vi "one plot adjustable to another.vi"(6 "country index":u16, 7 "SA data":T1, 8 "Countries (in)":string[](array[string]), 9 "US data":T1, 10 "deaths CSV":string[][](array[string]), 11 "cases CSV":string[][](array[string])) -> ()   [LabVIEW 2019]
panel:
  out "XY Graph":T2(graph)
  in  "Country 2":u16(ring) items=["Afghanistan", "Albania", "Algeria", "Andorra", "Angola", "Antigua and Barbuda", "Argentina", "Armenia", "Australia, Australian Capital Territory", "Australia, New South Wales", "Australia, Northern Territory", "Australia, Queensland", "Australia, South Australia", "Australia, Tasmania", "Australia, Victoria", "Australia, Western Australia", "Austria", "Azerbaijan", "Bahamas", "Bahrain", "Bangladesh", "Barbados", "Belarus", "Belgium", "Benin", "Bhutan", "Bolivia", "Bosnia and Herzegovina", "Brazil", "Brunei", "Bulgaria", "Burkina Faso", "Cabo Verde", "Cambodia", "Cameroon", "Canada, Alberta", "Canada, British Columbia", "Canada, Grand Princess", "Canada, Manitoba", "Canada, New Brunswick", "Canada, Newfoundland and Labrador", "Canada, Nova Scotia", "Canada, Ontario", "Canada, Prince Edward Island", "Canada, Quebec", "Canada, Saskatchewan", "Central African Republic", "Chad", "Chile", "China, Anhui", "China, Beijing", "China, Chongqing", "China, Fujian", "China, Gansu", "China, Guangdong", "China, Guangxi", "China, Guizhou", "China, Hainan", "China, Hebei", "China, Heilongjiang", "China, Henan", "China, Hong Kong", "China, Hubei", "China, Hunan", "China, Inner Mongolia", "China, Jiangsu", "China, Jiangxi", "China, Jilin", "China, Liaoning", "China, Macau", "China, Ningxia", "China, Qinghai", "China, Shaanxi", "China, Shandong", "China, Shanghai", "China, Shanxi", "China, Sichuan", "China, Tianjin", "China, Tibet", "China, Xinjiang", "China, Yunnan", "China, Zhejiang", "Colombia", "Congo (Brazzaville)", "Congo (Kinshasa)", "Costa Rica", "Cote d'Ivoire", "Croatia", "Diamond Princess", "Cuba", "Cyprus", "Czechia", "Denmark, Faroe Islands", "Denmark, Greenland", "Denmark", "Djibouti", "Dominican Republic", "Ecuador", "Egypt", "El Salvador", "Equatorial Guinea", "Eritrea", "Estonia", "Eswatini", "Ethiopia", "Fiji", "Finland", "France, French Guiana", "France, French Polynesia", "France, Guadeloupe", "France, Mayotte", "France, New Caledonia", "France, Reunion", "France, Saint Barthelemy", "France, St Martin", "France, Martinique", "France", "Gabon", "Gambia", "Georgia", "Germany", "Ghana", "Greece", "Guatemala", "Guinea", "Guyana", "Haiti", "Holy See", "Honduras", "Hungary", "Iceland", "India", "Indonesia", "Iran", "Iraq", "Ireland", "Israel", "Italy", "Jamaica", "Japan", "Jordan", "Kazakhstan", "Kenya", "Korea South", "Kuwait", "Kyrgyzstan", "Latvia", "Lebanon", "Liberia", "Liechtenstein", "Lithuania", "Luxembourg", "Madagascar", "Malaysia", "Maldives", "Malta", "Mauritania", "Mauritius", "Mexico", "Moldova", "Monaco", "Mongolia", "Montenegro", "Morocco", "Namibia", "Nepal", "Netherlands, Aruba", "Netherlands, Curacao", "Netherlands, Sint Maarten", "Netherlands", "New Zealand", "Nicaragua", "Niger", "Nigeria", "North Macedonia", "Norway", "Oman", "Pakistan", "Panama", "Papua New Guinea", "Paraguay", "Peru", "Philippines", "Poland", "Portugal", "Qatar", "Romania", "Russia", "Rwanda", "Saint Lucia", "Saint Vincent and the Grenadines", "San Marino", "Saudi Arabia", "Senegal", "Serbia", "Seychelles", "Singapore", "Slovakia", "Slovenia", "Somalia", "South Africa", "Spain", "Sri Lanka", "Sudan", "Suriname", "Sweden", "Switzerland", "Taiwan*", "Tanzania", "Thailand", "Togo", "Trinidad and Tobago", "Tunisia", "Turkey", "Uganda", "Ukraine", "United Arab Emirates", "United Kingdom, Bermuda", "United Kingdom, Cayman Islands", "United Kingdom, Channel Islands", "United Kingdom, Gibraltar", "United Kingdom, Isle of Man", "United Kingdom, Montserrat", "United Kingdom", "Uruguay", "US", "Uzbekistan", "Venezuela", "Vietnam", "Zambia", "Zimbabwe", "Canada, Diamond Princess", "Dominica", "Grenada", "Mozambique", "Syria", "Timor-Leste", "Belize", "Laos", "Libya", "West Bank and Gaza", "Guinea-Bissau", "Mali", "Saint Kitts and Nevis", "Canada, Northwest Territories", "Canada, Yukon", "Kosovo", "Burma", "United Kingdom, Anguilla", "United Kingdom, British Virgin Islands", "United Kingdom, Turks and Caicos Islands", "MS Zaandam", "Botswana", "Burundi", "Sierra Leone", "Netherlands, \"Bonaire Sint Eustatius and Saba\"", "Malawi", "United Kingdom, Falkland Islands (Malvinas)", "France, Saint Pierre and Miquelon", "South Sudan", "Western Sahara", "Sao Tome and Principe", "Yemen", "Comoros", "Tajikistan", "Lesotho", "Australia", "Western Europe", "Latin America", "Africa", "China", "US and Canada", "US - Northeast", "US - Midwest", "US - South", "US - West", "Scandinavia (excl Sweden)", "Middle East", "Global", "American Samoa", "Guam", "Northern Mariana Islands", "Puerto Rico", "Virgin Islands", "Alabama", "Alaska", "Arizona", "Arkansas", "California", "Colorado", "Connecticut", "Delaware", "Florida", "Georgia", "Hawaii", "Idaho", "Illinois", "Indiana", "Iowa", "Kansas", "Kentucky", "Louisiana", "Maine", "Maryland", "Massachusetts", "Michigan", "Minnesota", "Mississippi", "Missouri", "Montana", "Nebraska", "Nevada", "New Hampshire", "New Jersey", "New Mexico", "New York", "North Carolina", "North Dakota", "Ohio", "Oklahoma", "Oregon", "Pennsylvania", "Rhode Island", "South Carolina", "South Dakota", "Tennessee", "Texas", "Utah", "Vermont", "Virginia", "Washington", "West Virginia", "Wisconsin", "Wyoming"]
  in  "Data":u16(ring) items=["cumulative cases", "new cases per day", "cumulative deaths", "new deaths per day"]
  in  "Days":u16=7
  in  "Moving average":bool
  in  "Country 1":u16(ring) items=["Afghanistan", "Albania", "Algeria", "Andorra", "Angola", "Antigua and Barbuda", "Argentina", "Armenia", "Australia, Australian Capital Territory", "Australia, New South Wales", "Australia, Northern Territory", "Australia, Queensland", "Australia, South Australia", "Australia, Tasmania", "Australia, Victoria", "Australia, Western Australia", "Austria", "Azerbaijan", "Bahamas", "Bahrain", "Bangladesh", "Barbados", "Belarus", "Belgium", "Benin", "Bhutan", "Bolivia", "Bosnia and Herzegovina", "Brazil", "Brunei", "Bulgaria", "Burkina Faso", "Cabo Verde", "Cambodia", "Cameroon", "Canada, Alberta", "Canada, British Columbia", "Canada, Grand Princess", "Canada, Manitoba", "Canada, New Brunswick", "Canada, Newfoundland and Labrador", "Canada, Nova Scotia", "Canada, Ontario", "Canada, Prince Edward Island", "Canada, Quebec", "Canada, Saskatchewan", "Central African Republic", "Chad", "Chile", "China, Anhui", "China, Beijing", "China, Chongqing", "China, Fujian", "China, Gansu", "China, Guangdong", "China, Guangxi", "China, Guizhou", "China, Hainan", "China, Hebei", "China, Heilongjiang", "China, Henan", "China, Hong Kong", "China, Hubei", "China, Hunan", "China, Inner Mongolia", "China, Jiangsu", "China, Jiangxi", "China, Jilin", "China, Liaoning", "China, Macau", "China, Ningxia", "China, Qinghai", "China, Shaanxi", "China, Shandong", "China, Shanghai", "China, Shanxi", "China, Sichuan", "China, Tianjin", "China, Tibet", "China, Xinjiang", "China, Yunnan", "China, Zhejiang", "Colombia", "Congo (Brazzaville)", "Congo (Kinshasa)", "Costa Rica", "Cote d'Ivoire", "Croatia", "Diamond Princess", "Cuba", "Cyprus", "Czechia", "Denmark, Faroe Islands", "Denmark, Greenland", "Denmark", "Djibouti", "Dominican Republic", "Ecuador", "Egypt", "El Salvador", "Equatorial Guinea", "Eritrea", "Estonia", "Eswatini", "Ethiopia", "Fiji", "Finland", "France, French Guiana", "France, French Polynesia", "France, Guadeloupe", "France, Mayotte", "France, New Caledonia", "France, Reunion", "France, Saint Barthelemy", "France, St Martin", "France, Martinique", "France", "Gabon", "Gambia", "Georgia", "Germany", "Ghana", "Greece", "Guatemala", "Guinea", "Guyana", "Haiti", "Holy See", "Honduras", "Hungary", "Iceland", "India", "Indonesia", "Iran", "Iraq", "Ireland", "Israel", "Italy", "Jamaica", "Japan", "Jordan", "Kazakhstan", "Kenya", "Korea South", "Kuwait", "Kyrgyzstan", "Latvia", "Lebanon", "Liberia", "Liechtenstein", "Lithuania", "Luxembourg", "Madagascar", "Malaysia", "Maldives", "Malta", "Mauritania", "Mauritius", "Mexico", "Moldova", "Monaco", "Mongolia", "Montenegro", "Morocco", "Namibia", "Nepal", "Netherlands, Aruba", "Netherlands, Curacao", "Netherlands, Sint Maarten", "Netherlands", "New Zealand", "Nicaragua", "Niger", "Nigeria", "North Macedonia", "Norway", "Oman", "Pakistan", "Panama", "Papua New Guinea", "Paraguay", "Peru", "Philippines", "Poland", "Portugal", "Qatar", "Romania", "Russia", "Rwanda", "Saint Lucia", "Saint Vincent and the Grenadines", "San Marino", "Saudi Arabia", "Senegal", "Serbia", "Seychelles", "Singapore", "Slovakia", "Slovenia", "Somalia", "South Africa", "Spain", "Sri Lanka", "Sudan", "Suriname", "Sweden", "Switzerland", "Taiwan*", "Tanzania", "Thailand", "Togo", "Trinidad and Tobago", "Tunisia", "Turkey", "Uganda", "Ukraine", "United Arab Emirates", "United Kingdom, Bermuda", "United Kingdom, Cayman Islands", "United Kingdom, Channel Islands", "United Kingdom, Gibraltar", "United Kingdom, Isle of Man", "United Kingdom, Montserrat", "United Kingdom", "Uruguay", "US", "Uzbekistan", "Venezuela", "Vietnam", "Zambia", "Zimbabwe", "Canada, Diamond Princess", "Dominica", "Grenada", "Mozambique", "Syria", "Timor-Leste", "Belize", "Laos", "Libya", "West Bank and Gaza", "Guinea-Bissau", "Mali", "Saint Kitts and Nevis", "Canada, Northwest Territories", "Canada, Yukon", "Kosovo", "Burma", "United Kingdom, Anguilla", "United Kingdom, British Virgin Islands", "United Kingdom, Turks and Caicos Islands", "MS Zaandam", "Botswana", "Burundi", "Sierra Leone", "Netherlands, \"Bonaire Sint Eustatius and Saba\"", "Malawi", "United Kingdom, Falkland Islands (Malvinas)", "France, Saint Pierre and Miquelon", "South Sudan", "Western Sahara", "Sao Tome and Principe", "Yemen", "Comoros", "Tajikistan", "Lesotho", "Australia", "Western Europe", "Latin America", "Africa", "China", "US and Canada", "US - Northeast", "US - Midwest", "US - South", "US - West", "Scandinavia (excl Sweden)", "Middle East", "Global", "American Samoa", "Guam", "Northern Mariana Islands", "Puerto Rico", "Virgin Islands", "Alabama", "Alaska", "Arizona", "Arkansas", "California", "Colorado", "Connecticut", "Delaware", "Florida", "Georgia", "Hawaii", "Idaho", "Illinois", "Indiana", "Iowa", "Kansas", "Kentucky", "Louisiana", "Maine", "Maryland", "Massachusetts", "Michigan", "Minnesota", "Mississippi", "Missouri", "Montana", "Nebraska", "Nevada", "New Hampshire", "New Jersey", "New Mexico", "New York", "North Carolina", "North Dakota", "Ohio", "Oklahoma", "Oregon", "Pennsylvania", "Rhode Island", "South Carolina", "South Dakota", "Tennessee", "Texas", "Utah", "Vermont", "Virginia", "Washington", "West Virginia", "Wisconsin", "Wyoming"]
  out "mortality rate":dbl
  in  "Up/Down increment size":dbl=5.0 min=0.01 max=10.0
  in  "Down":bool
  in  "Up":bool
  out "Days ahead":i32
  in  "right":bool
  in  "left":bool
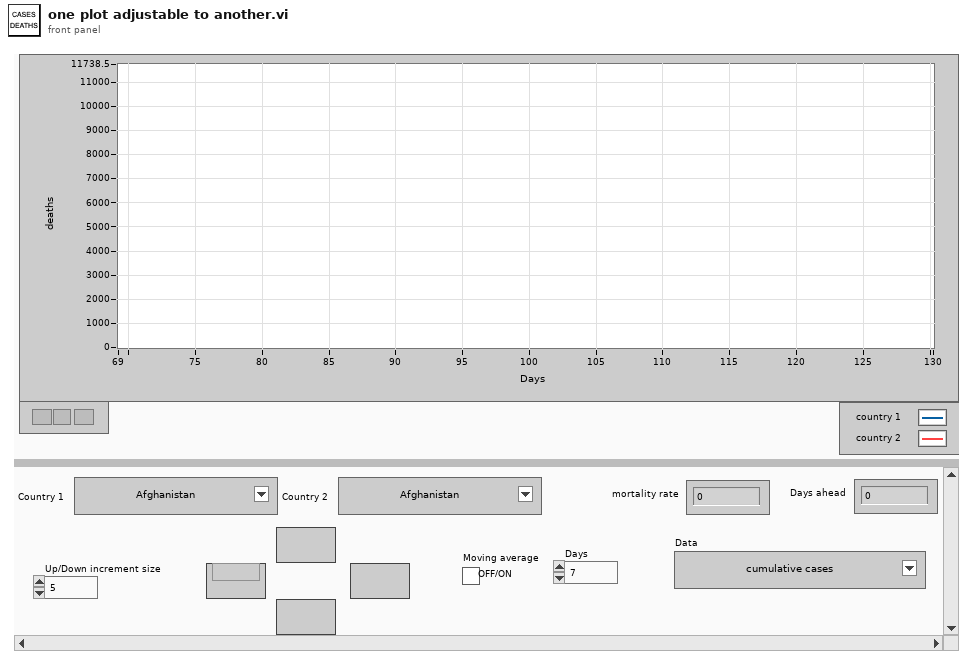
[diagram p1: front panel]
types:
  T1 = cluster{"cumulative deaths":i32[][], "deaths per day":i32[][], "case per day":i32[][], "cumulative cases":i32[][]}
  T2 = cluster{"cases days":i32[], "moving average array":dbl[]}[]
  T3 = cluster{"array index":i32[], "moving average array":dbl[]}
  T4 = cluster{"array index":i32[], "moving average array":dbl[]}[]
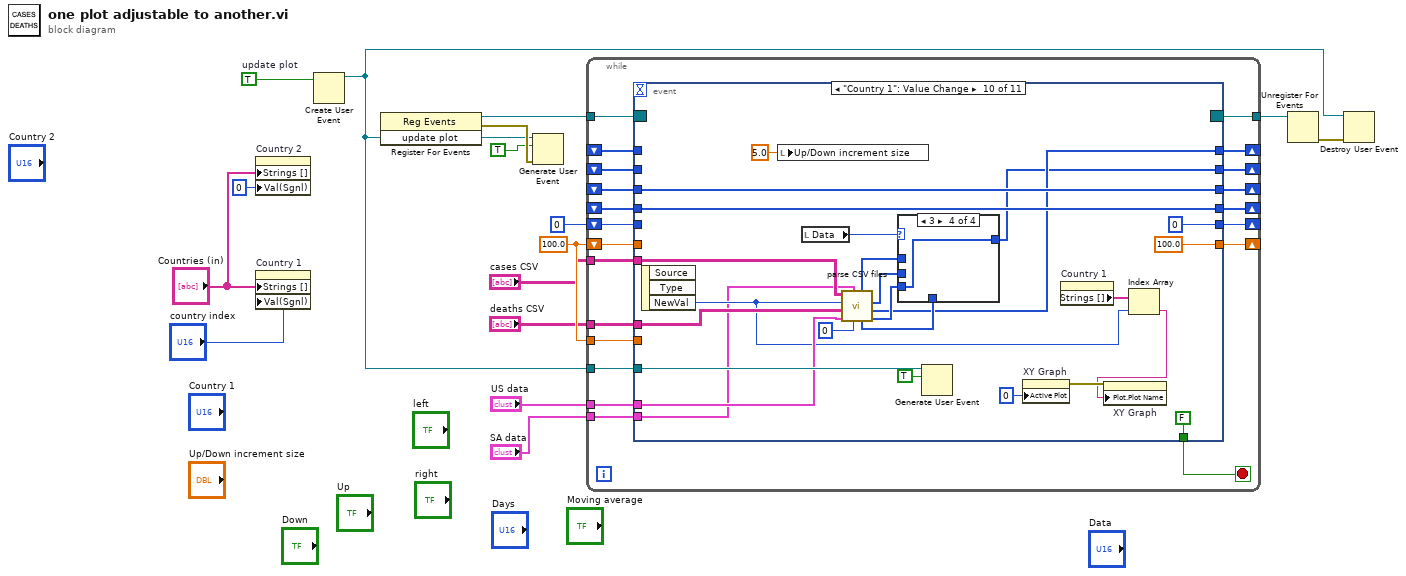
[diagram p0: block diagram]
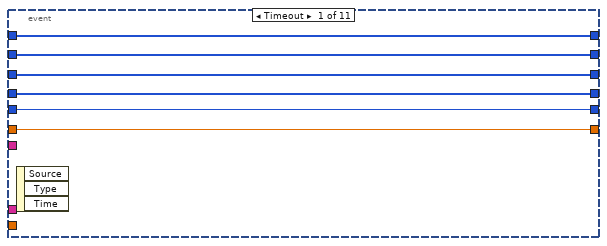
[diagram p2: hidden frame]
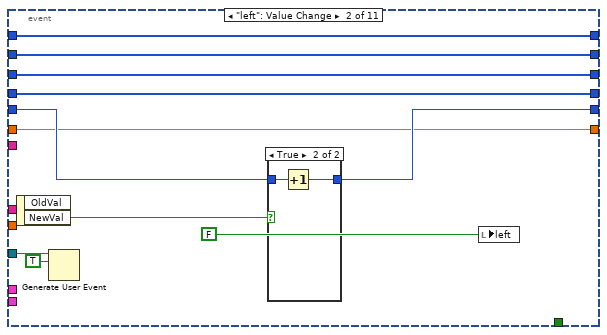
[diagram p3: hidden frame]
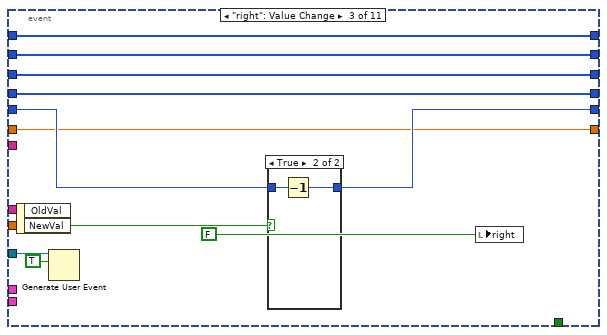
[diagram p5: hidden frame]
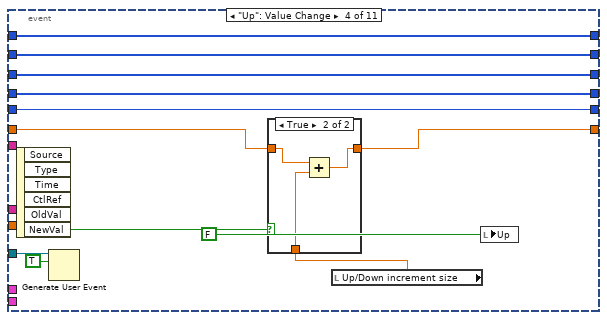
[diagram p7: hidden frame]
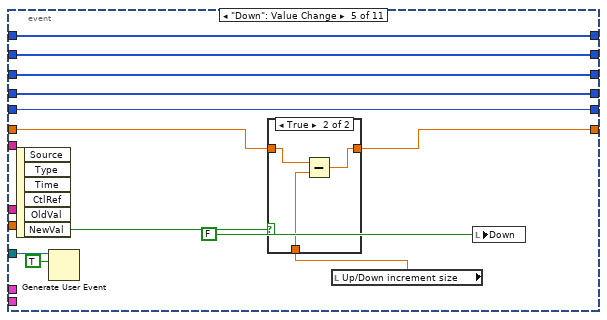
[diagram p9: hidden frame]
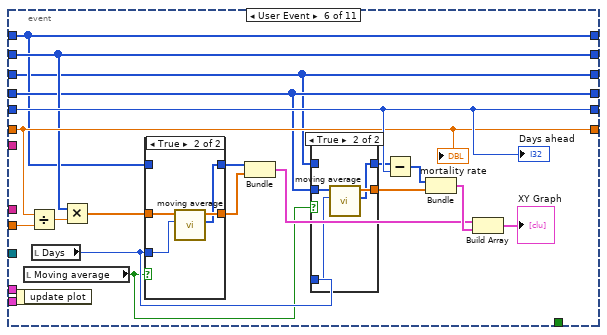
[diagram p11: hidden frame]
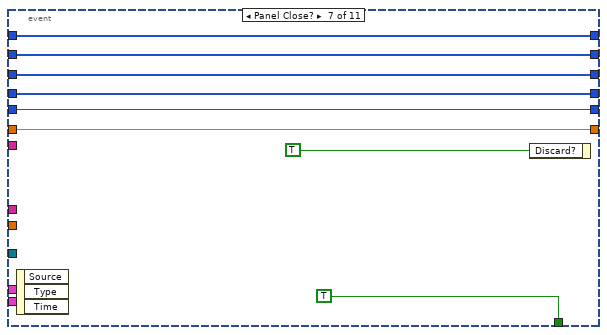
[diagram p14: hidden frame]
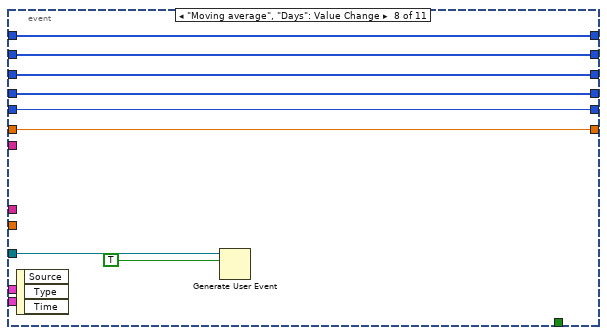
[diagram p15: hidden frame]
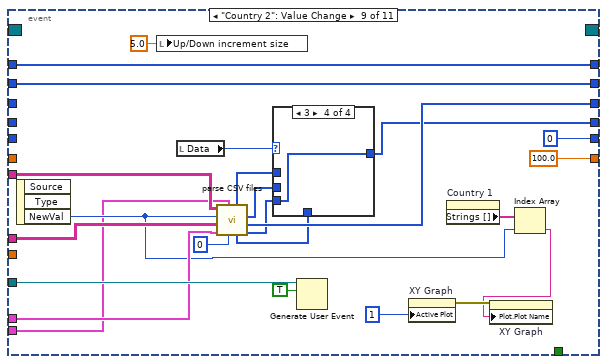
[diagram p16: hidden frame]
diagram:
  w12 = 100.0
  w14 = TRUE  # update plot
  n1 = property on="Country 2" class="Ring (strict)"("Strings []"="Countries (in)", "Val(Sgnl)"=u16 0 ("Value (Signaling)")) -> ()  [unwired: 2 in, 2 out]
  n2 = property on="Country 1" class="Ring (strict)"("Strings []"="Countries (in)", "Val(Sgnl)"="country index") -> ()  [unwired: 2 in, 2 out]
  n3 = Create User Event(user event datatype=w14) -> (user event=w8:refnum<user-event>)  [unwired: 1 in, 1 out]
  n4 = register-events(w8) -> (reference out=w15:refnum<event-registration>, error out=w13:errorcluster)  [unwired: 2 in]
  n5 = Generate User Event(user event=w8, event data cluster=TRUE ("event data"), error in=w13) -> ()  [unwired: 1 in, 2 out]
  n6 = while {
    shift-right: [w33] -> _
    shift-left: _ -> [w37]
    shift-right: [w32] -> _
    shift-left: _ -> [w36]
    shift-right: [w30] -> _
    shift-left: _ -> [w35]
    shift-right: [w31] -> _
    shift-left: _ -> [w34]
    shift-right: [w28] -> _
    shift-left: 0 -> [w29]
    tunnel: w15 -> [w27]
    tunnel: w8 -> [w26]
    shift-right: [w24] -> _
    shift-left: w12 -> [w25]
    tunnel: w12 -> [w23]
    tunnel: [w21] -> w10
    tunnel: "cases CSV" -> [w20]
    tunnel: "deaths CSV" -> [w19]
    tunnel: "US data" -> [w18]
    tunnel: "SA data" -> [w17]
    stop <- w22 stop-if-true
    n7 = event shown="[9] \"Country 1\": Value Change" {
      selector: w27 -> [_ _ _ _ _ _ _ _ _ _ _]
      dyn-events: [_ _ _ _ _ _ _ _ _ _ _] -> w21
      timeout: _ -> [_ _ _ _ _ _ _ _ _ _ _]
      tunnel: w37 -> [w43 w54 w68 w83 w99 w108 w135 w143 w164 _ _]
      tunnel: w36 -> [w42 w53 w67 w82 w98 w114 w142 w150 w163 _ w214]
      tunnel: w35 -> [w40 w52 w66 w81 w97 w111 w140 w148 _ w188 w212]
      tunnel: w34 -> [w41 w51 w65 w80 w96 w106 w141 w149 _ w189 w213]
      tunnel: [w43 w54 w68 w83 w99 w108 w135 w143 w164 w187 _] -> w33
      tunnel: [w42 w53 w67 w82 w98 w114 w142 w150 w163 w186 w214] -> w32
      tunnel: [w41 w51 w65 w80 w96 w106 w141 w149 w165 w189 w213] -> w31
      tunnel: [w40 w52 w66 w81 w97 w111 w140 w148 w157 w188 w212] -> w30
      tunnel: w29 -> [w39 w50 w64 w75 w91 w116 w139 w147 _ _ w211]
      tunnel: [w39 w49 w63 w75 w91 w116 w139 w147 0 0 w211] -> w28
      tunnel: w26 -> [_ w47 w62 w79 w95 _ _ w145 w171 w200 _]
      tunnel: w25 -> [w38 w44 w58 w74 w90 w115 w138 w146 _ _ w210]
      tunnel: [w38 w44 w58 w72 w88 w115 w138 w146 100.0 100.0 w210] -> w24
      tunnel: w23 -> [_ _ _ _ _ w118 _ _ _ _ _]
      tunnel: [_ _ _ _ _ _ TRUE _ _ FALSE _] -> w22
      tunnel: w20 -> [_ _ _ _ _ _ _ _ w168 w197 _]
      tunnel: w19 -> [_ _ _ _ _ _ _ _ w167 w196 _]
      tunnel: w18 -> [_ _ _ _ _ _ _ _ w166 w195 _]
      tunnel: w17 -> [_ _ _ _ _ _ _ _ w151 w179 _]
      event Timeout {
        n8 = event-data() -> ()  [unwired: 1 in, 3 out]
      }
      event "left": Value Change {
        n9 = event-data() -> ("NewVal"=w48:bool)  [unwired: 1 in, 1 out]
        n10 = Generate User Event(user event=w47, event data cluster=TRUE ("event data")) -> ()  [unwired: 2 in, 2 out]
        n11 = case shown="True" w48 {
          tunnel: w50 -> [w55 w57]
          tunnel: [w55 w56] -> w49
          frame False {
          }
          frame True {
            n12 = Increment(x=w57) -> (x+1=w56:i32)
          }
        }
        n13 = local write "left"(FALSE ("Previous Button")) -> ()
      }
      event "right": Value Change {
        n14 = event-data() -> ("NewVal"=w59:bool)  [unwired: 1 in, 1 out]
        n15 = Generate User Event(user event=w62, event data cluster=TRUE ("event data")) -> ()  [unwired: 2 in, 2 out]
        n16 = case shown="True" w59 {
          tunnel: w64 -> [w69 w71]
          tunnel: [w69 w70] -> w63
          frame False {
          }
          frame True {
            n17 = Decrement(x=w71) -> (x-1=w70:i32)
          }
        }
        n18 = local write "right"(FALSE ("Previous Button")) -> ()
      }
      event "Up": Value Change {
        n19 = event-data() -> ("NewVal"=w76:bool)  [unwired: 1 in, 5 out]
        n20 = Generate User Event(user event=w79, event data cluster=TRUE ("event data")) -> ()  [unwired: 2 in, 2 out]
        n21 = local read "Up/Down increment size"() -> (w73:dbl)
        n22 = case shown="True" w76 {
          tunnel: w74 -> [w84 w87]
          tunnel: [w84 w86] -> w72
          tunnel: w73 -> [_ w85]
          frame False {
          }
          frame True {
            n23 = Add(x=w87, y=w85) -> (x+y=w86:dbl)
          }
        }
        n24 = local write "Up"(FALSE ("Previous Button")) -> ()
      }
      event "Down": Value Change {
        n25 = event-data() -> ("NewVal"=w92:bool)  [unwired: 1 in, 5 out]
        n26 = Generate User Event(user event=w95, event data cluster=TRUE ("event data")) -> ()  [unwired: 2 in, 2 out]
        n27 = local read "Up/Down increment size"() -> (w89:dbl)
        n28 = case shown="True" w92 {
          tunnel: w90 -> [w100 w103]
          tunnel: [w100 w102] -> w88
          tunnel: w89 -> [_ w101]
          frame False {
          }
          frame True {
            n29 = Subtract(x=w103, y=w101) -> (x-y=w102:dbl)
          }
        }
        n30 = local write "Down"(FALSE ("Previous Button")) -> ()
      }
      event User Event {
        n31 = event-data() -> ()  [unwired: 1 in, 1 out]
        n32 = local read "Moving average"() -> (w104:bool)
        n33 = Divide(x=w115, y=w118) -> (x/y=w117:dbl)
        n34 = local read "Days"() -> (w109:u16)
        n35 = Multiply(x=w114, y=w117) -> (x*y=w113:dbl[])
        n36 = case shown="True" w104 {
          tunnel: w113 -> [w129 w134]
          tunnel: [w129 w133] -> w112
          tunnel: w109 -> [_ w132]
          tunnel: w108 -> [w130 _]
          tunnel: [w130 w131] -> w107
          frame False {
          }
          frame True {
            n37 = call "moving average.vi"("average over x points"=w132, "Array"=w134) -> ("array index"=w131:i32[], "moving average array"=w133:dbl[])  [unwired: 8 in]
          }
        }
        n38 = Bundle("array index"=w107, "moving average array"=w112) -> (w121:T3)  [unwired: 1 in]
        n39 = case shown="True" w104 {
          tunnel: w111 -> [w123 w128]
          tunnel: [w123 w127] -> w110
          tunnel: w109 -> [_ w126]
          tunnel: w106 -> [w124 _]
          tunnel: [w124 w125] -> w105
          frame False {
          }
          frame True {
            n40 = call "moving average.vi"("average over x points"=w126, "Array"=w128) -> ("array index"=w125:i32[], "moving average array"=w127:dbl[])  [unwired: 8 in]
          }
        }
        n41 = Subtract(x=w105, y=w116) -> (x-y=w120:i32[])
        n42 = Bundle(w120, "moving average array"=w110) -> (w122:cluster{i32[], "moving average array":dbl[]})  [unwired: 1 in]
        n43 = Build Array(w121, w122) -> (→"XY Graph":T4)
        "Days ahead" <- w116
        "mortality rate" <- w115
      }
      event Panel Close? {
        n44 = event-data() -> ()  [unwired: 1 in, 3 out]
        n45 = event-data("Discard?"=TRUE) -> ()  [unwired: 1 in, 1 out]
      }
      event "Moving average", "Days": Value Change {
        n46 = event-data() -> ()  [unwired: 1 in, 3 out]
        n47 = Generate User Event(user event=w145, event data cluster=TRUE ("event data")) -> ()  [unwired: 2 in, 2 out]
      }
      event "Country 2": Value Change {
        n48 = event-data() -> ("NewVal"=w154:u16)  [unwired: 1 in, 2 out]
        n49 = local write "Up/Down increment size"(5.0 ("Up/Down increment size")) -> ()
        n50 = local read "Data"() -> (w158:u16)
        n51 = call "parse CSV files.vi"("threshold cases"=u32 0, "SA data"=w151, "US data"=w166, "deaths CSV"=w167, "country index"=w154, "cases CSV"=w168) -> ("new deaths per day"=w161:i32[], "days"=w165:i32[], "new cases per day"=w162:i32[], "cumulative cases"=w160:i32[], "cumulative deaths"=w159:i32[])  [unwired: 1 out]
        n52 = case shown="3" w158 {
          tunnel: w162 -> [_ w176 _ _]
          tunnel: w161 -> [_ _ _ w178]
          tunnel: w160 -> [w175 _ _ _]
          tunnel: w159 -> [_ _ w177 _]
          tunnel: [w175 w176 w177 w178] -> w157
          frame 0, Default {
          }
          frame 1 {
          }
          frame 2 {
          }
          frame 3 {
          }
        }
        n53 = Generate User Event(user event=w171, event data cluster=TRUE ("event data")) -> ()  [unwired: 2 in, 2 out]
        n54 = property on="XY Graph" class="XYGraph (strict)"("Active Plot"=u32 1) -> (error out=w156:errorcluster)  [unwired: 2 in, 1 out]
        n55 = property on="Country 1" class="Ring (strict)"() -> ("Strings []"=w155:string[])  [unwired: 2 in, 2 out]
        n56 = Index Array(array=w155, index=w154) -> (element=w153:string)
        n57 = property on="XY Graph" class="XYGraph (strict)"(error in=w156, "Plot.Plot Name"=w153) -> ()  [unwired: 1 in, 2 out]
      }
      event "Country 1": Value Change {
        n58 = event-data() -> ("NewVal"=w181:u16)  [unwired: 1 in, 2 out]
        n59 = local write "Up/Down increment size"(5.0 ("Up/Down increment size")) -> ()
        n60 = local read "Data"() -> (w190:u16)
        n61 = call "parse CSV files.vi"("threshold cases"=u32 0, "SA data"=w179, "US data"=w195, "deaths CSV"=w196, "country index"=w181, "cases CSV"=w197) -> ("new deaths per day"=w193:i32[], "days"=w187:i32[], "new cases per day"=w194:i32[], "cumulative cases"=w192:i32[], "cumulative deaths"=w191:i32[])  [unwired: 1 out]
        n62 = case shown="3" w190 {
          tunnel: w194 -> [_ w205 _ _]
          tunnel: w193 -> [_ _ _ w207]
          tunnel: w192 -> [w204 _ _ _]
          tunnel: w191 -> [_ _ w206 _]
          tunnel: [w204 w205 w206 w207] -> w186
          frame 0, Default {
          }
          frame 1 {
          }
          frame 2 {
          }
          frame 3 {
          }
        }
        n63 = Generate User Event(user event=w200, event data cluster=TRUE ("event data")) -> ()  [unwired: 2 in, 2 out]
        n64 = property on="XY Graph" class="XYGraph (strict)"("Active Plot"=u32 0) -> (error out=w184:errorcluster)  [unwired: 2 in, 1 out]
        n65 = property on="Country 1" class="Ring (strict)"() -> ("Strings []"=w182:string[])  [unwired: 2 in, 2 out]
        n66 = Index Array(array=w182, index=w181) -> (element=w180:string)
        n67 = property on="XY Graph" class="XYGraph (strict)"(error in=w184, "Plot.Plot Name"=w180) -> ()  [unwired: 1 in, 2 out]
      }
      event "Data": Value Change {
        n68 = event-data() -> ()  [unwired: 1 in, 6 out]
        n69 = local read "Country 1"() -> (w209:u16)
        n70 = local read "Country 2"() -> (w208:u16)
        n71 = property on="Country 2" class="Ring (strict)"("Val(Sgnl)"=w208) -> ()  [unwired: 2 in, 2 out]
        n72 = property on="Country 1" class="Ring (strict)"("Val(Sgnl)"=w209) -> ()  [unwired: 2 in, 2 out]
      }
    }
  }
  n73 = Unregister For Events(event registration refnum=w10) -> (error out=w9:errorcluster)  [unwired: 1 in]
  n74 = Destroy User Event(user event=w8, error in=w9) -> ()  [unwired: 1 out]
